vi "Get Daemon Error.vi"(8 "error in (no error)":errorcluster, 11 "Modbus slave in":refnum<class "Modbus Slave.lvclass">) -> (0 "error out":errorcluster, 2 "daemon error":errorcluster, 3 "Modbus slave out":refnum<class "Modbus Slave.lvclass">)   [LabVIEW 2015, in "Modbus Slave.lvclass"]
doc: "<B>Daemon Error</B> returns the error information about the daemon."
uses:
  <vilib>/Modbus/slave/Modbus Slave.lvclass
  <vilib>/Modbus/slave/Modbus Slave.lvclass/Modbus Slave.ctl
  <vilib>/Modbus/subvis/Protocol/Interfaces/Network Slave/Network Slave.lvclass
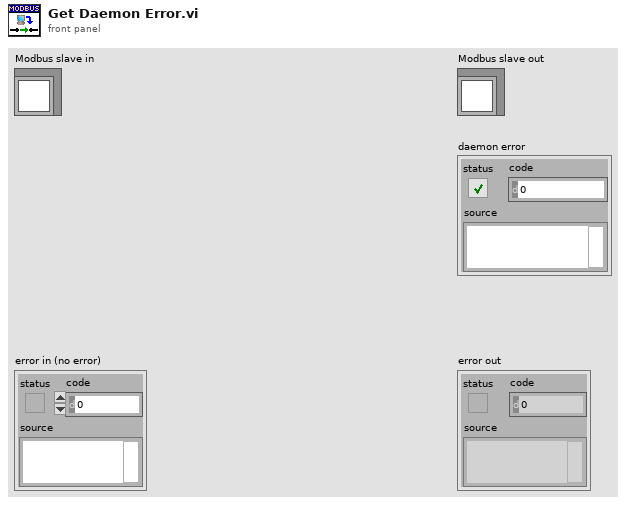
[diagram p1: front panel]
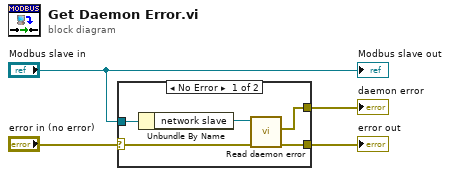
[diagram p0: block diagram]
diagram:
  n1 = case shown="No Error" "error in (no error)" {
    selector: "error in (no error)" -> [w5 w10]
    tunnel: [w9 w10] -> w4
    tunnel: "Modbus slave in" -> [w8 _]
    tunnel: [w7 _] -> w2
    frame No Error {
      n2 = Unbundle By Name(w8) -> ("network slave"=w6:refnum<class "Network Slave.lvclass">)
      n3 = call <vilib>:"Read daemon error.vi"("error in (no error)"=w5, "network slave in"=w6) -> ("error out"=w9:errorcluster, "daemon error"=w7:errorcluster)  [unwired: 7 in, 1 out]
    }
    frame Error {
    }
  }
  "error out" <- w4
  "daemon error" <- w2
  "Modbus slave out" <- "Modbus slave in"
